vi "test_Export Instrument Addon Config with Error.vi"(8 "error in (no error)":errorcluster, 11 "TestCase in":refnum<class "Instrument Addon Scripting API Custom Device Unit Tests.lvclass">) -> (0 "error out":errorcluster, 3 "TestCase out":refnum<class "Instrument Addon Scripting API Custom Device Unit Tests.lvclass">)   [LabVIEW 2019, in "Instrument Addon Scripting API Custom Device Unit Tests.lvclass"]
uses:
  Instrument Addon Scripting API Custom Device Unit Tests.lvclass
  <vilib>/addons/_JKI Toolkits/VI Tester/TestCase.llb/TestCase.lvclass
  APIs/Scripting API/Instrument Addon Scripting API.lvlib
  NationalInstruments.VeriStand.SystemDefinitionAPI
  <vilib>/NI VeriStand/Custom Device Tools/Custom Device Utility Library/Custom Device Utility Library.lvlib
  Addon/Addon Shared/SubVIs/Constants.vi
  Addon/Addon Shared/Instrument Addon Shared.lvlib
  <vilib>/NI VeriStand/Custom Device Tools/Custom Device Utility Library/NI VeriStand - Search for Item by GUID.vi
  C:/Program Files (x86)/National Instruments/LabVIEW 2019/vi.lib/addons/_JKI Toolkits/VI Tester/TestCase.llb/TestCase.lvclass
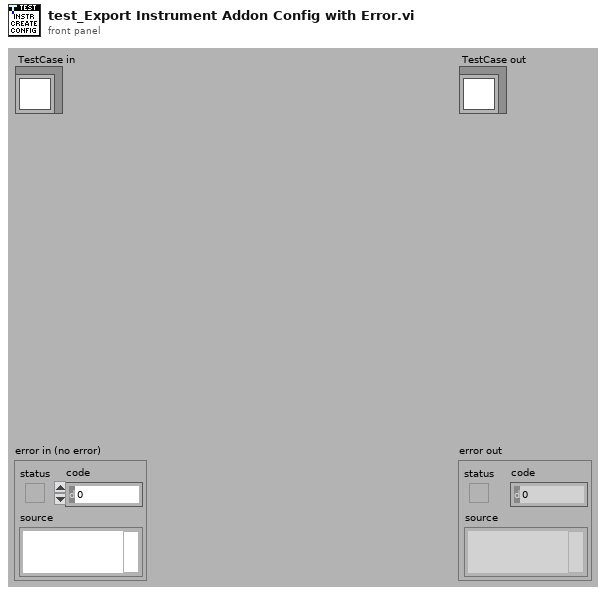
[diagram p1: front panel]
types:
  T1 = typedef "Custom Device API.lvlib/Custom Device Item Ref.ctl" = u64
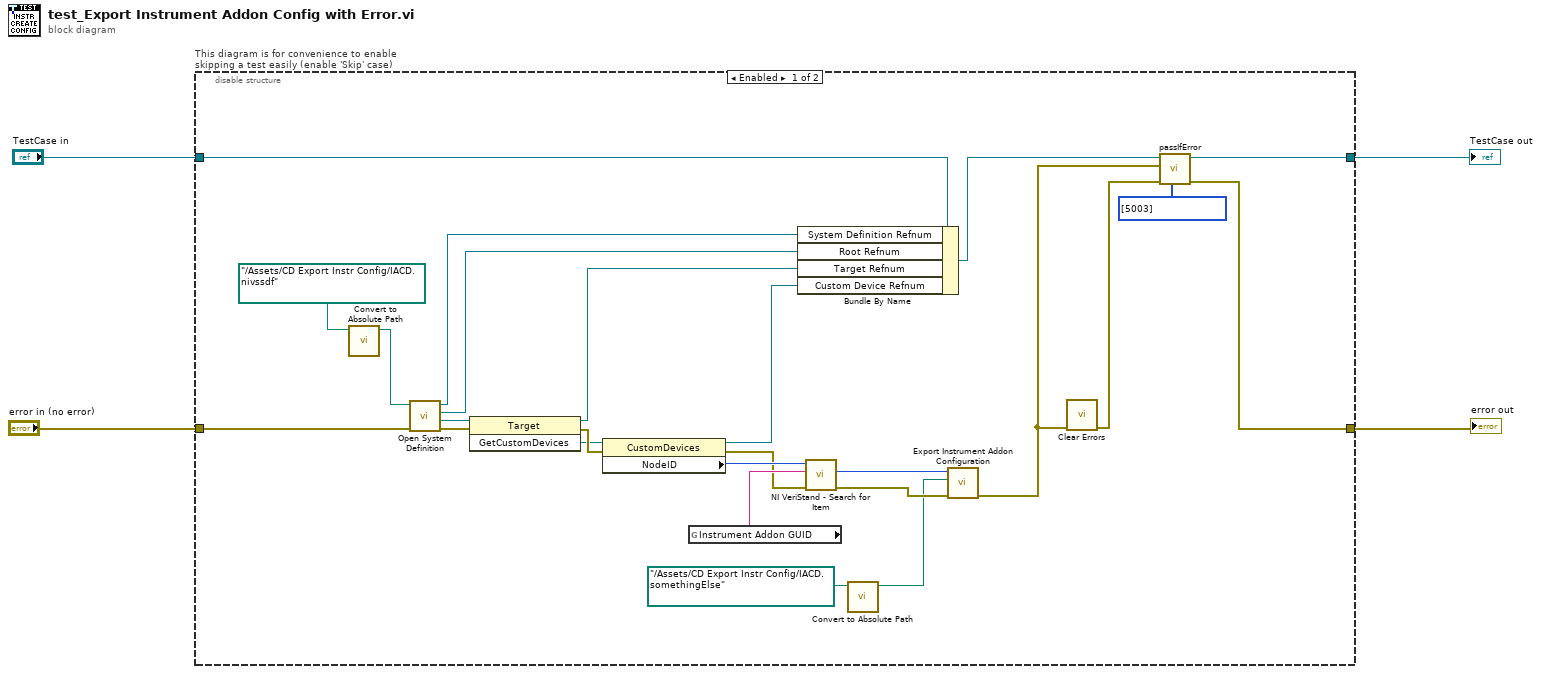
[diagram p0: block diagram]
diagram:
  n1 = disable-structure "This diagram is for convenience to enable skipping a test easily (enable 'Skip' case)" shown="Enabled" {
    disable-tunnel: "TestCase in" -> [w10 w33]
    disable-tunnel: [w14 w31] -> w1
    disable-tunnel: [w12 w32] -> w3
    disable-tunnel: "error in (no error)" -> [w29 w30]
    frame Enabled {
      n2 = call "Convert to Absolute Path.vi"("System Definition File"=path "../Assets/CD Export Instr Config/IACD.nivssdf" ("SDF file")) -> ("Absolute Path"=w27:path)  [unwired: 10 in]
      n3 = call "Open System Definition.vi"("error in (no error)"=w29, "System Definition File"=w27) -> ("error out"=w23:errorcluster, "Target Refnum"=w22:refnum<k24>, "Root Refnum"=w7:refnum<k24>, "System Definition Refnum"=w8:refnum<k24>)  [unwired: 6 in]
      n4 = invoke class="Target" method="GetCustomDevices"(reference=w22, error in=w23) -> (reference out=w6:refnum<k24>, error out=w25:errorcluster, "GetCustomDevices"=w24:refnum<k24>)  [unwired: 1 in]
      n5 = property class="CustomDevices"(reference=w24, error in=w25) -> (reference out=w5:refnum<k24>, error out=w19:errorcluster, "NodeID"=w21:u64)
      n6 = global read "Constants.vi" "Instrument Addon GUID"() -> (w20:string)
      n7 = Bundle By Name(cluster=w10, "System Definition Refnum"=w8, "Root Refnum"=w7, "Target Refnum"=w6, "Custom Device Refnum"=w5) -> (w9:refnum<class "Instrument Addon Scripting API Custom Device Unit Tests.lvclass">)
      n8 = call-poly <vilib>:"NI VeriStand - Search for Item.vi"("error in"=w19, "Item GUID"=w20, "Section Ref in"=w21) -> ("error out"=w18:errorcluster, "Item Ref"=w17:T1)  [unwired: 5 in, 2 out]
      n9 = call "Convert to Absolute Path.vi"("System Definition File"=path "../Assets/CD Export Instr Config/IACD.somethingElse" ("SDF file")) -> ("Absolute Path"=w16:path)  [unwired: 10 in]
      n10 = call "Export Instrument Addon Configuration.vi"("error in (no error)"=w18, "export file path"=w16, "instrument addon refnum in"=w17) -> ("error out"=w15:errorcluster)  [unwired: 7 in, 1 out]
      n11 = call <vilib>:"Clear Errors.vi"("error in (no error)"=w15) -> ("error out"=w11:errorcluster)  [unwired: 5 in, 1 out]
      n12 = call-dynamic "passIfError.vi"("passing error codes (default = any error code)"=i32[] [5003], "error in (no error)"=w11, "error"=w15, "TestCase in"=w9) -> ("error out"=w12:errorcluster, "TestCase out"=w14:refnum<class "Instrument Addon Scripting API Custom Device Unit Tests.lvclass">)  [unwired: 6 in]
    }
    frame Disabled {
      # "skip test result while test is under development"
      n13 = call <vilib>:"skip.vi"("error in (no error)"=w30, "TestCase in"=w33) -> ("error out"=w32:errorcluster, "TestCase out"=w31:refnum<class "Instrument Addon Scripting API Custom Device Unit Tests.lvclass">)  [unwired: 8 in]
    }
  }
  "error out" <- w3
  "TestCase out" <- w1
